vi "send trigger.vi"(8 "error in (no error)":errorcluster, 11 "TDK-Lambda Z in":refnum<class "TDK-Lambda Z.lvclass">) -> (0 "error out":errorcluster, 3 "TDK-Lambda Z out":refnum<class "TDK-Lambda Z.lvclass">)   [LabVIEW 2013, in "TDK-Lambda Z.lvclass"]
uses:
  TDK-Lambda Z.lvclass
  OnOffTypeDef.ctl
  TDK-Lambda Z.lvclass/TDK-Lambda Z.ctl
  TDK-Lambda Z.lvlib
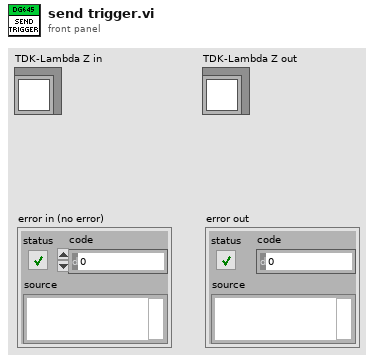
[diagram p1: front panel]
types:
  T1 = typedef "OnOffTypeDef.ctl" = enum16{"off", "on"}
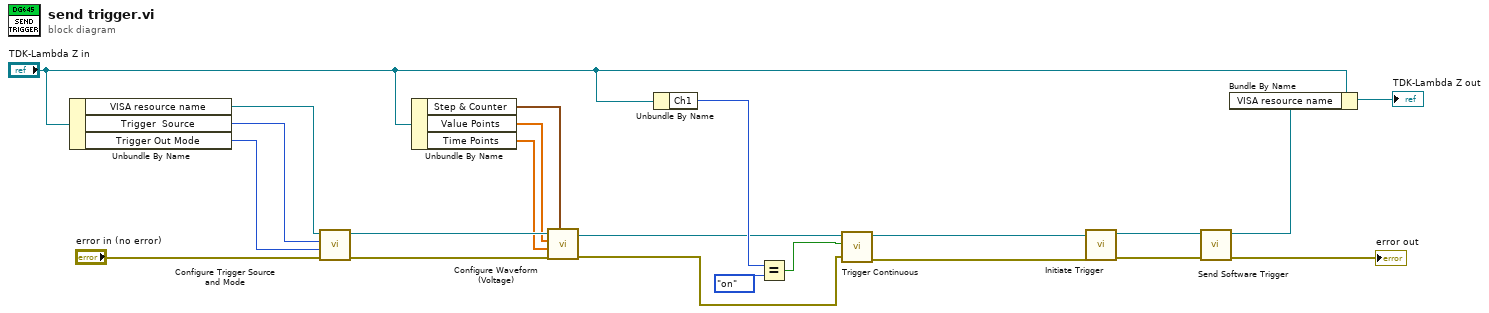
[diagram p0: block diagram]
diagram:
  n1 = Unbundle By Name("TDK-Lambda Z in") -> ("VISA resource name"=w19:refnum<visa-resource-name>, "Trigger  Source"=w18:u16, "Trigger Out Mode"=w17:u16)
  n2 = call "Configure Trigger Source and Mode.vi"("error in (no error)"="error in (no error)", "Trigger Out Mode (0: Off)"=w17, "Trigger  Source (0: External)"=w18, "VISA resource name"=w19) -> ("error out"=w15:errorcluster, "VISA resource name out"=w14:refnum<visa-resource-name>)  [unwired: 6 in]
  n3 = Unbundle By Name("TDK-Lambda Z in") -> ("Step & Counter"=w13:cluster{"Step (0: Once)":u16, "Counter (1)":i32}, "Value Points"=w12:dbl[], "Time Points"=w11:dbl[])
  n4 = call "Configure Waveform (Voltage).vi"("Step & Counter"=w13, "error in (no error)"=w15, "Time Points"=w11, "Value Points"=w12, "VISA resource name"=w14) -> ("error out"=w8:errorcluster, "VISA resource name out"=w7:refnum<visa-resource-name>)  [unwired: 5 in]
  n5 = Unbundle By Name("TDK-Lambda Z in") -> ("Ch1"=w9:T1)
  n6 = Equal?(x=w9, y=OnOffTypeDef."on") -> (x = y?=w22:bool)
  n7 = call "Trigger Continuous.vi"("error in (no error)"=w8, "Continuous Trigger (F: Off)"=w22, "VISA resource name"=w7) -> ("error out"=w6:errorcluster, "VISA resource name out"=w5:refnum<visa-resource-name>)  [unwired: 7 in]
  n8 = call "Initiate Trigger.vi"("error in (no error)"=w6, "VISA resource name"=w5) -> ("error out"=w3:errorcluster, "VISA resource name out"=w4:refnum<visa-resource-name>)  [unwired: 8 in]
  n9 = call "Send Software Trigger.vi"("error in (no error)"=w3, "VISA resource name"=w4) -> ("error out"=→"error out":errorcluster, "VISA resource name out"=w2:refnum<visa-resource-name>)  [unwired: 8 in]
  n10 = Bundle By Name(cluster="TDK-Lambda Z in", "VISA resource name"=w2) -> (→"TDK-Lambda Z out":refnum<class "TDK-Lambda Z.lvclass">)
